vi "Hardware Subpanels.vi"   [LabVIEW 2020]
uses:
  <vilib>/Utility/miscctls.llb/LVPositionTypeDef.ctl
  Plugin Servers/Controller Array/Controller Array.lvclass/Controller Array.ctl
  Plugin Servers/Controller/Generic Plugin.lvclass/Generic Plugin.ctl
  Plugin Servers/Controller/Generic Plugin.lvclass
  Plugin Servers/Controller Array/Controller Array.lvclass
types:
  T1 = typedef "LVPositionTypeDef.ctl" = cluster{"Left":i32, "Top":i32}
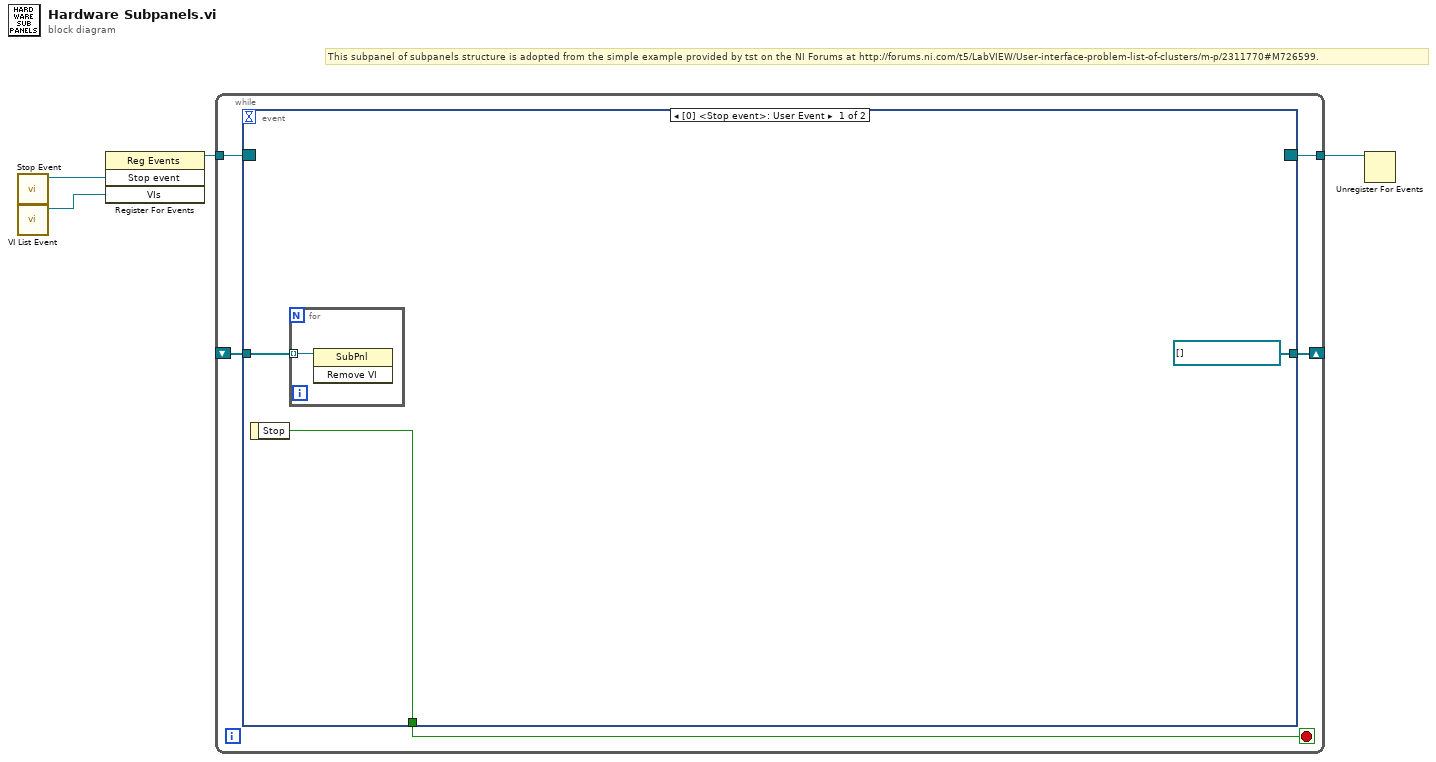
[diagram p0: block diagram]
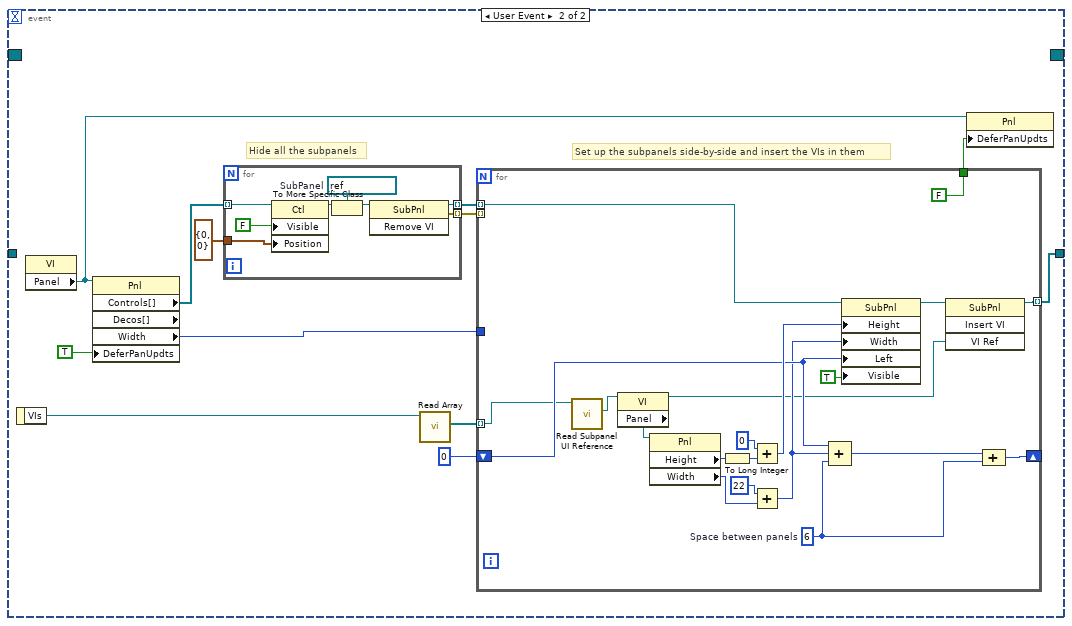
[diagram p2: hidden frame]
diagram:
  # "This subpanel of subpanels structure is adopted from the simple example provided by tst on the NI Forums at http://forums.ni.com/t5/LabVIEW/User-interface-problem-list-of-clusters/m-p/2311770#M726599."
  n1 = call "Stop Event.vi"() -> ("Stop event"=w2:refnum<user-event>)  [unwired: 11 out]
  n2 = call "VI List Event.vi"() -> ("VIs"=w1:refnum<user-event>)  [unwired: 11 in]
  n3 = register-events(w2, w1) -> (reference out=w4:refnum<event-registration>)  [unwired: 2 in, 1 out]
  n4 = while {
    tunnel: w4 -> [w9]
    tunnel: [w8] -> w3
    shift-right: [w6] -> _
    shift-left: _ -> [w5]
    stop <- w7 stop-if-true
    n5 = event shown="[0] <Stop event>: User Event" {
      selector: w9 -> [_ _]
      dyn-events: [_ _] -> w8
      timeout: _ -> [_ _]
      tunnel: [w10 _] -> w7
      tunnel: [refnum<vi>[] [] w21] -> w6
      tunnel: w5 -> [w12 _]
      event User Event {
        n6 = event-data() -> ("Stop"=w10:bool)  [unwired: 1 out]
        n7 = for {
          tunnel: w12 -> [w13] mode=indexing
          n8 = invoke class="SubPnl" method="Remove VI"(reference=w13) -> ()  [unwired: 2 in, 3 out]
        }
      }
      event User Event {
        # "Set up the subpanels side-by-side and insert the VIs in them"
        # "Hide all the subpanels"
        n9 = event-data() -> ("VIs"=w15:refnum<class "Controller Array.lvclass">)  [unwired: 1 out]
        n10 = property class="VI"() -> ("Panel"=w18:refnum<vi>)  [unwired: 2 in, 2 out]
        n11 = property class="Pnl" props=["Controls[]", "Decos[]", "Width", "DeferPanUpdts"](reference=w18, "DeferPanUpdts"=TRUE ("Defer Panel Updates")) -> ("Controls[]"=w23:refnum<vi>[], "Width"=w25:u32)  [unwired: 1 in, 3 out]
        n12 = for {
          tunnel: w23 -> [w33] mode=indexing
          tunnel: T1 {"Left"=0, "Top"=0} ("Position") -> [w31]
          tunnel: [w27] -> w17 mode=indexing
          tunnel: [w26] -> w16 mode=indexing
          w30 = refnum<vi> refnum  # SubPanel
          n13 = property class="Ctl"(reference=w33, "Visible"=FALSE, "Position"=w31) -> (reference out=w28:refnum<vi>)  [unwired: 1 in, 1 out]
          n14 = To More Specific Class(target class=w30, reference=w28) -> (specific class reference=w29:refnum<vi>)  [unwired: 1 in, 1 out]
          n15 = invoke class="SubPnl" method="Remove VI"(reference=w29) -> (reference out=w26:refnum<vi>, error out=w27:errorcluster)  [unwired: 2 in, 1 out]
        }
        n16 = call "Read Array.vi"("Controller Array in"=w15) -> ("Array"=w14:refnum<class "Generic Plugin.lvclass">[])  [unwired: 8 in, 2 out]
        n17 = for {
          shift-right: [w50] -> _
          shift-left: 0 -> [w39]
          tunnel: [w45] -> w21 mode=indexing
          tunnel: w25 -> [_]
          tunnel: [FALSE ("Defer Panel Updates")] -> w19
          tunnel: w17 -> [_] mode=indexing
          tunnel: w16 -> [w40] mode=indexing
          tunnel: w14 -> [w34] mode=indexing
          w51 = 6  # Space between panels
          n18 = call "Read Subpanel UI Reference.vi"("controller in"=w34) -> ("Subpanel UI Reference"=w35:refnum<vi>)  [unwired: 8 in, 2 out]
          n19 = property class="VI"(reference=w35) -> (reference out=w36:refnum<vi>, "Panel"=w37:refnum<vi>)  [unwired: 1 in, 1 out]
          n20 = property class="Pnl"(reference=w37) -> ("Height"=w49:u32, "Width"=w41:u32)  [unwired: 1 in, 2 out]
          n21 = To Long Integer(number=w49) -> (32bit integer=w46:i32)
          n22 = Add(x=0, y=w46) -> (x+y=w48:i32)
          n23 = Add(x=u32 22, y=w41) -> (x+y=w38:u32)
          n24 = Compound Arithmetic op=ADD(w39, w38, w51) -> (w52:u32)
          n25 = property class="SubPnl"(reference=w40, "Height"=w48, "Width"=w38, "Left"=w39, "Visible"=TRUE) -> (reference out=w53:refnum<vi>)  [unwired: 1 in, 1 out]
          n26 = invoke class="SubPnl" method="Insert VI"(reference=w53, "VI Ref"=w36) -> (reference out=w45:refnum<vi>)  [unwired: 2 in, 3 out]
          n27 = Compound Arithmetic op=ADD(w52, w51) -> (w50:u32)
        }
        n28 = property class="Pnl"(reference=w18, "DeferPanUpdts"=w19) -> ()  [unwired: 1 in, 2 out]
      }
    }
  }
  n29 = Unregister For Events(event registration refnum=w3) -> ()  [unwired: 1 in, 1 out]
